vi "Remove_Plug_Ins_etc.vi"(1 "Input String":string) -> (0 "Output string":string)   [LabVIEW 2010]
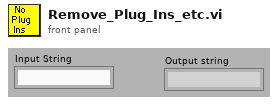
[diagram p1: front panel]
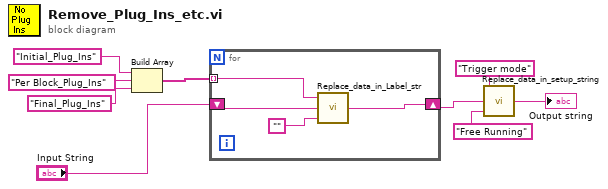
[diagram p0: block diagram]
diagram:
  n1 = Build Array("Initial_Plug_Ins", "Per Block_Plug_Ins", "Final_Plug_Ins") -> (w4:string[])
  n2 = for {
    shift-right: [w11] -> w7
    shift-left: "Input String" -> [w12]
    tunnel: w4 -> [w13] mode=indexing
    n3 = call "Replace_data_in_Label_str.vi"("New data string"="", "Input string"=w12, "Variable name"=w13) -> ("Appended string"=w11:string)
  }
  n4 = call "Replace_data_in_setup_string.vi"("New data string"="Free Running", "Input string"=w7, "Variable name"="Trigger mode") -> ("Appended string"=→"Output string":string)
